vi "Memory.Pointer.Read.Safe.0D.Bool.vi"(8 "error in (no error)":errorcluster, 9 "offset (0)":u64 format="%d bytes", 10 "value in":bool, 11 "pointer in":refnum<class "Memory.Pointer.lvclass">) -> (0 "error out":errorcluster, 1 "offset out":u64 format="%d bytes", 2 "value out":bool, 3 "pointer out":refnum<class "Memory.Pointer.lvclass">)   [LabVIEW 2016, in "Memory.lvlib" / "Memory.Pointer.lvclass"]
doc: "Reads the contents of the address specified by <b>pointer + offset</b> into <b>value</b>.\n\n<b>Note:</b> This VI is <b>safe</b>.\n\nSafe means that this function evaluates the size parameter of <b>pointer</b> to ensure that is inbounds of allocated memory before peforming a memory read/write. Reading/writing more data to a pointer than it has allocated can corrupt or crash LabVIEW."
uses:
  Memory.Pointer.lvclass
  Memory.Pointer.lvclass/Memory.Pointer.ctl
  Memory.Pointer.Get Address.vi
  Memory.Pointer.Errors.vi
  Memory.Pointer.Errors.Null Pointer.vi
  Memory.Pointer.Errors.Out of Bounds.vi
  Memory.Pointer.Get Size.vi
  Memory.Pointer.Errors.Create Error.vi
  Submodules/SEH/Source/VIs/Static Error Handling.Source Buffer.Write.String.vi
  Memory.Pointer.Errors.Write Pointer Size.vi
  Submodules/SEH/Source/VIs/Static Error Handling.Source Buffer.Write.Numeric.Scalar.Base10.vi
  Submodules/SEH/Source/VIs/Static Error Handling.Source Buffer.Write.Numeric.Scalar.Base10 (U64).vi
  Submodules/SEH/Source/VIs/Static Error Handling.Error Cluster Constant.vi
  Submodules/SEH/Source/VIs/Static Error Handling.Error Cluster Constant (256B).vi
  Submodules/SEH/Source/VIs/Static Error Handling.Parameters.Status.Set.vi
  Submodules/SEH/Source/VIs/Static Error Handling.Parameters.Code.Set.vi
  Submodules/SEH/Source/VIs/Static Error Handling.Parameters.VI Source.Set.vi
  Constants/Memory.Constants.vi
  Constants/Memory.Constants.Library Name.vi
  Memory.Pointer.Errors.Get Info.vi
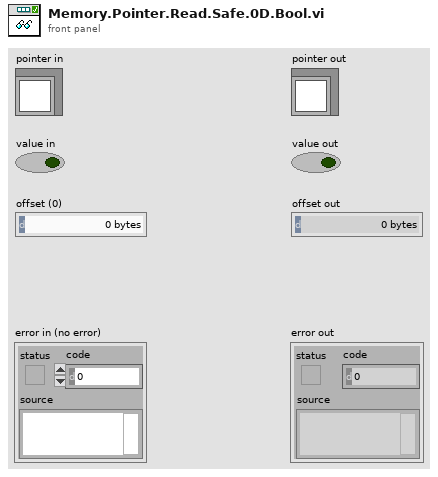
[diagram p1: front panel]
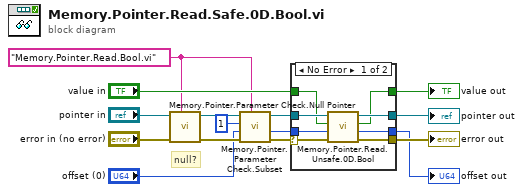
[diagram p0: block diagram]
diagram:
  w4 = "Memory.Pointer.Read.Bool.vi" ("source vi name")
  # "null?"
  n1 = call "Memory.Pointer.Parameter Check.Null Pointer.vi"("source vi name"=w4, "error in (no error)"="error in (no error)", "Pointer in"="pointer in") -> ("error out"=w6:errorcluster, "Pointer out"=w5:refnum<class "Memory.Pointer.lvclass">)  [unwired: 7 in]
  n2 = call "Memory.Pointer.Parameter Check.Subset.vi"("source vi name"=w4, "error in (no error)"=w6, "offset (0)"="offset (0)", "length"=u64 1 ("y"), "Pointer in"=w5) -> ("error out"=w10:errorcluster, "offset out"=w3:u64, "Pointer out"=w12:refnum<class "Memory.Pointer.lvclass">)  [unwired: 3 in, 1 out]
  n3 = case shown="No Error" w10 {
    selector: w10 -> [w19 w25]
    tunnel: w12 -> [w23 w27]
    tunnel: [w22 w27] -> w15
    tunnel: [w21 w26] -> w14
    tunnel: "value in" -> [w20 w26]
    tunnel: [w18 w25] -> w9
    tunnel: w3 -> [w17 w24]
    tunnel: [w16 w24] -> w1
    frame No Error {
      n4 = call "Memory.Pointer.Read.Unsafe.0D.Bool.vi"("error in (no error)"=w19, "offset (0)"=w17, "value in"=w20, "pointer in"=w23) -> ("error out"=w18:errorcluster, "offset out"=w16:u64, "value out"=w21:bool, "pointer out"=w22:refnum<class "Memory.Pointer.lvclass">)  [unwired: 4 in]
    }
    frame Error {
    }
  }
  "error out" <- w9
  "pointer out" <- w15
  "value out" <- w14
  "offset out" <- w1
